vi "sendInfoLoopToLoop.vi"(11 "scan info":T1) -> (0 "num empty spaces for commands":u32, 1 "num successful commands looped":u32, 3 "numLoopToLoopErrors":u32)   [LabVIEW 2010]
uses:
  scan_command.ctl
  <vilib>/rvi/DataTransferAndStorage/Container/XNode/niFpgaContainer.xnode
  <vilib>/rvi/FIFO/Fifo_Resource/nirvififoEmulationSetSize.vi
  <vilib>/rvi/DataTransferAndStorage/Container/Common/niFpgaContainerGetUniqueNameForEmu.vi
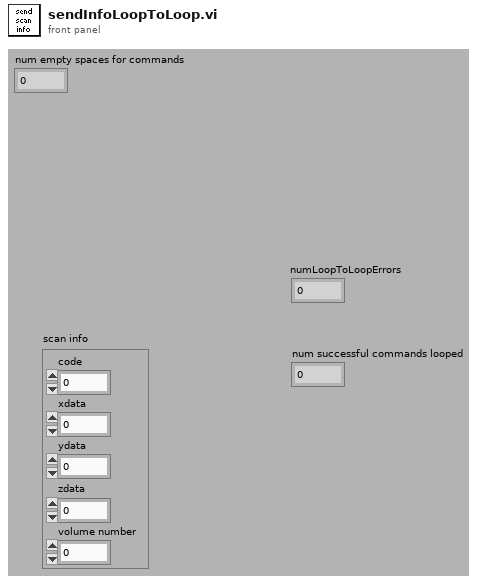
[diagram p1: front panel]
types:
  T1 = typedef "scan_command.ctl" = cluster{"code":i32, "xdata":i32, "ydata":i32, "zdata":i32, "volume number":i32}
  T2 = cluster{"code":i32, "xdata":i32, "ydata":i32, "zdata":i32, "volume number":i32}
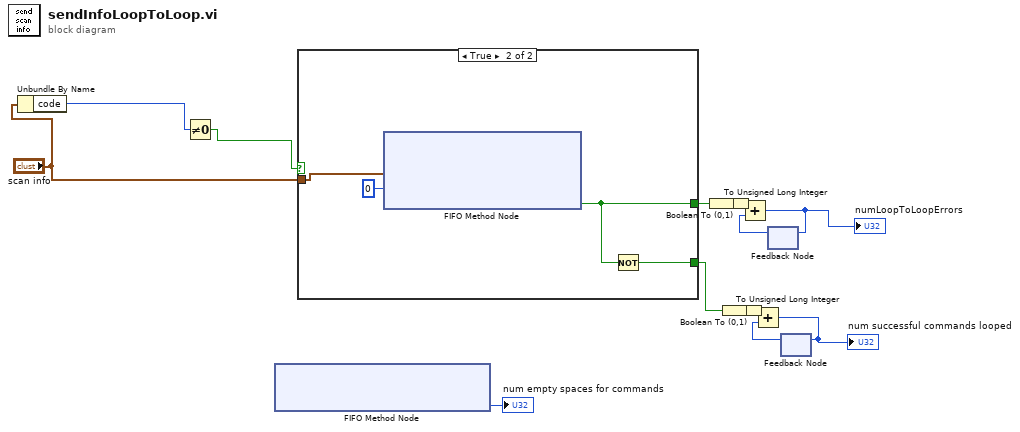
[diagram p0: block diagram]
diagram:
  n1 = Unbundle By Name("scan info") -> ("code"=w8:i32)
  n2 = Not Equal To 0?(x=w8) -> (x != 0?=w1:bool)
  n3 = xnode ("FIFO Method Node")() -> ("Number of Elements to Write"=→"num empty spaces for commands":u32)  [unwired: 1 in, 1 out]
  n4 = case shown="True" w1 {
    tunnel: "scan info" -> [_ w17]
    tunnel: [_ w16] -> w14
    tunnel: [_ w15] -> w3
    frame False {
    }
    frame True {
      n5 = xnode ("FIFO Method Node")("Element"=w17, "Timeout"=0) -> ("Timed Out?"=w16:bool)  [unwired: 1 in, 1 out]
      n6 = Not(x=w16) -> (.not. x?=w15:bool)
    }
  }
  n7 = Boolean To (0,1)(Boolean=w14) -> (0, 1=w11:i16)
  n8 = Boolean To (0,1)(Boolean=w3) -> (0, 1=w5:i16)
  n9 = To Unsigned Long Integer(number=w11) -> (unsigned 32bit integer=w10:u32)
  n10 = To Unsigned Long Integer(number=w5) -> (unsigned 32bit integer=w4:u32)
  n11 = feedback #1() -> (w12:u32)  [unwired: 1 in]
  n12 = Add(x=w10, y=w12) -> (x+y=w13:u32)
  "numLoopToLoopErrors" <- w13
  n13 = feedback-in #1(w13) -> ()
  n14 = feedback #2() -> (w6:u32)  [unwired: 1 in]
  n15 = Add(x=w4, y=w6) -> (x+y=w7:u32)
  "num successful commands looped" <- w7
  n16 = feedback-in #2(w7) -> ()
